vi "Konwersja_temperatury.vi"(8 "Precyzja":sgl min=0 max=6 step=1, 9 "?":bool, 10 "Rezystancja":dbl, 11 "Skala temperatury":bool) -> (2 "Numeric":dbl format="%#_14g", 3 "String":string, 4 "Nieprawid³owa \nkonwersja":bool)   [LabVIEW 2020]
panel:
  # "Czujnik"
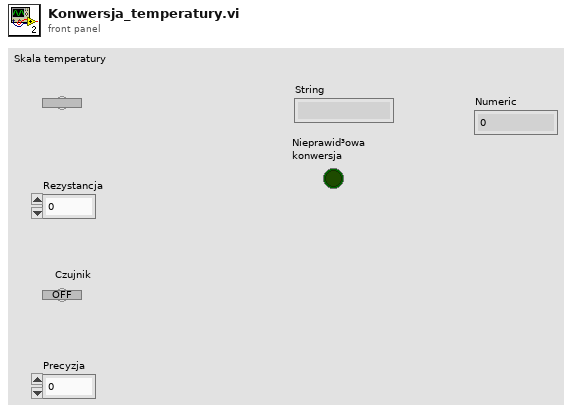
[diagram p1: front panel]
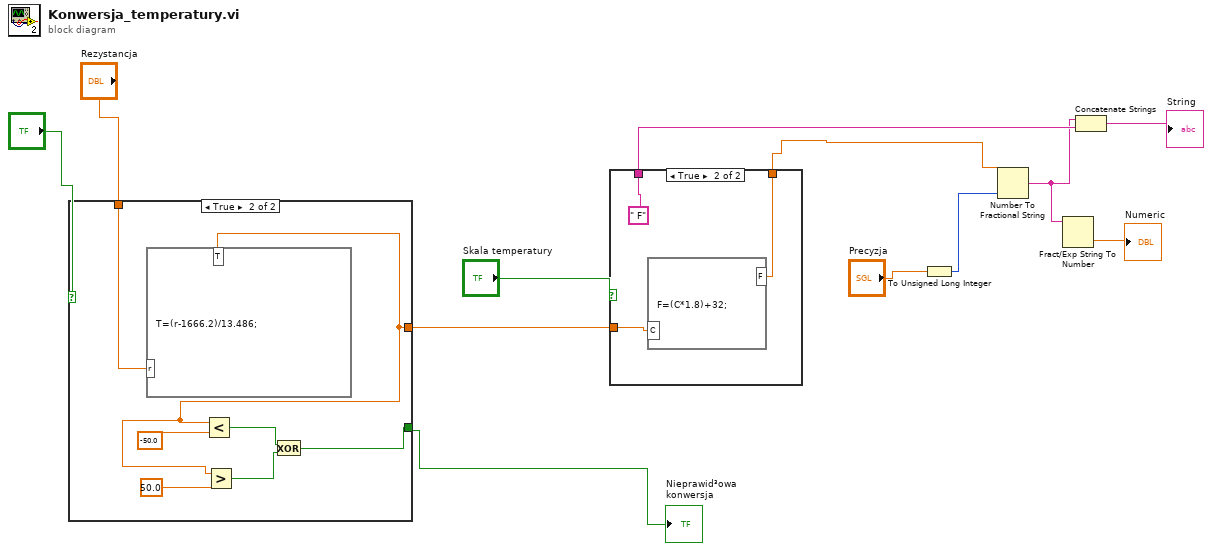
[diagram p0: block diagram]
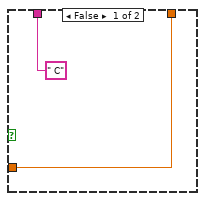
[diagram p2: hidden frame]
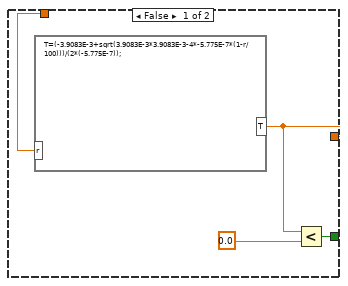
[diagram p3: hidden frame]
diagram:
  n1 = case shown="True" "?" {
    tunnel: "Rezystancja" -> [w16 w23]
    tunnel: [w15 w21] -> w9
    tunnel: [w13 w17] -> w10
    frame False {
      n2 = formula code="T=(-3.9083E-3+sqrt(3.9083E-3*3.9083E-3-4*-5.775E-7*(1-r/100)))/(2*(-5.775E-7));"("r"=w16) -> ("T"=w15:dbl)
      n3 = Less?(x=w15, y=0.0) -> (x < y?=w13:bool)
    }
    frame True {
      n4 = formula code="T=(r-1666.2)/13.486;"("r"=w23) -> ("T"=w21:dbl)
      n5 = Less?(x=w21, y=-50.0) -> (x < y?=w19:bool)
      n6 = Greater?(x=w21, y=50.0) -> (0:w18:bool)
      n7 = Exclusive Or(1:w18, 2:w19) -> (0:w17:bool)
    }
  }
  "Nieprawid³owa \nkonwersja" <- w10
  n8 = case shown="True" "Skala temperatury" {
    tunnel: [w25 w28] -> w5
    tunnel: w9 -> [w25 w27]
    tunnel: [" C" " F"] -> w11
    frame False {
    }
    frame True {
      n9 = formula code="F=(C*1.8)+32;"("C"=w27) -> ("F"=w28:dbl)
    }
  }
  n10 = To Unsigned Long Integer(number="Precyzja") -> (unsigned 32bit integer=w3:u32)
  n11 = Number To Fractional String(number=w5, precision (6)=w3) -> (F-format string=w2:string)  [unwired: 2 in]
  n12 = Fract/Exp String To Number(string=w2) -> (number=→"Numeric":dbl)  [unwired: 3 in, 1 out]
  n13 = Concatenate Strings(w2, w11) -> (→"String":string)
